vi "dfd_NStage MRate Response with Overall.vi"(4 "interpolated factors":i32[](array[numeric]), 5 "type (FLP)":enum16{"FLP", "FXP"}(ring), 6 "fs [Hz]":dbl, 7 "# freq bins (auto)":i32, 8 "error in (no error)":errorcluster, 9 "magnitude":u16(ring) items=["Linear", "dB", "Zero phase"], 10 "phase view":T1, 11 "multirate filters in":T2[](array[typedef]) {"mMRate_SumWl" min=1 max=32 step=1; "mMRate_InputIwl" min=1 max=32 step=1; "mMRate_GainWl" min=1 max=32 step=1; "mMRate_OutputWl" min=1 max=32 step=1; "mMRate_InputWl" min=1 max=32 step=1; "mMRate_CoefWl" min=1 max=32 step=1; "mMRate_Mode" items=["Default"=-1, "No Rate Change"=0, "Interpolation"=1, "Decimation"=2, "Interpolated"=3, "Rational"=4]}) -> (0 "error out":errorcluster, 2 "phase":cluster{dbl, "df":dbl, "phase":dbl[]}[](array[cluster]), 3 "mag":cluster{dbl, "df":dbl, "magnitude":dbl[]}[](array[cluster]))   [LabVIEW 2017, in "NI_DigFilterLicensed.lvlib"]
uses:
  <vilib>/addons/Digital Filter Design/NI_DigFilterLicensed.lvlib
  <vilib>/addons/Digital Filter Design/_Objects.llb/DFD Multirate Filter Obj.ctl
  <vilib>/addons/Digital Filter Design/_Objects.llb/DFD Multirate Mode.ctl
  <vilib>/addons/Digital Filter Design/_Objects.llb/DFD Coef Norm Type.ctl
  <vilib>/addons/Digital Filter Design/_Objects.llb/DFD Round-off Mode.ctl
  <vilib>/addons/Digital Filter Design/_Objects.llb/DFD FXP MRate Multiply Mode.ctl
  <vilib>/addons/Digital Filter Design/_Objects.llb/DFD Phase Setting.ctl
  <vilib>/Analysis/2dsp.llb/1D Convolution (DBL).vi
  <vilib>/Analysis/NI_AALPro.lvlib
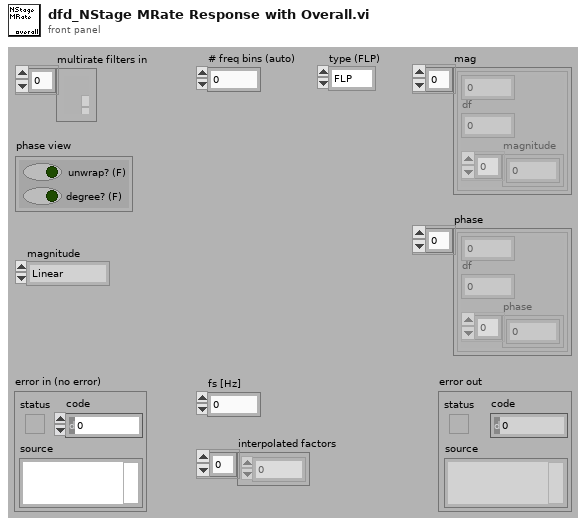
[diagram p1: front panel]
types:
  T1 = typedef "NI_DigFilterLicensed.lvlib/DFD Phase Setting.ctl" = cluster{"unwrap? (F)":bool, "degree? (F)":bool}
  T2 = typedef "NI_DigFilterLicensed.lvlib/DFD Multirate Filter Obj.ctl" = cluster{"mMRate_Structure":enum16{"CIC", "FIR", "IIR", "Lattice"}, "mMRate_Mode":T3, "mMRate_Factor":i32, "mMRate_FIRParams":cluster{"mMRate_FIR_H":dbl[], "mMRate_FIR_IsNyquist?":bool, "mMRate_FIR_IsSymmetric?":bool}, "mMRate_CICParams":cluster{"mMRate_CIC_#Stage":i32, "mMRate_CIC_Lag":i32, "mMRate_CIC_Type":enum16{"Lowpass", "Highpass"}}, "mMRate_Order":i32, "mMRate_Version":string, "mMRate_Comments":string, "mMRate_RationalFactor":cluster{"mMRate_L":i32, "mMRate_M":i32}, "mMRate_Fs":dbl, "mMRate_Quantized?":bool, "mMRate_QFilterGain":dbl, "mMRate_CoefWl":i16, "mMRate_Scaling":cluster{"mMRate_ScaleByPowerOf2?":bool, "mMRate_ScaleType":T4}, "mMRate_InputWl":i16, "mMRate_OutputWl":i16, "mMRate_OutputMode":T5, "mMRate_MultMode":T6, "mMRate_BitPruning":bool, "mMRate_GainWl":i16, "mMRate_OutputFwl":i16, "mMRate_SumIwl":i16, "mMRate_InputIwl ":i16, "mMRate_SumWl":i16, "mMRate_CoefIwl":i16}
  T3 = typedef "NI_DigFilterLicensed.lvlib/DFD Multirate Mode.ctl" = i16
  T4 = typedef "NI_DigFilterLicensed.lvlib/DFD Coef Norm Type.ctl" = enum16{"No Norm", "Time Domain 1-Norm", "Time Domain 2-Norm", "Time Domain Inf-Norm"}
  T5 = typedef "NI_DigFilterLicensed.lvlib/DFD Round-off Mode.ctl" = enum16{"Nearest", "Truncation"}
  T6 = typedef "NI_DigFilterLicensed.lvlib/DFD FXP MRate Multiply Mode.ctl" = enum16{"Truncated", "Full"}
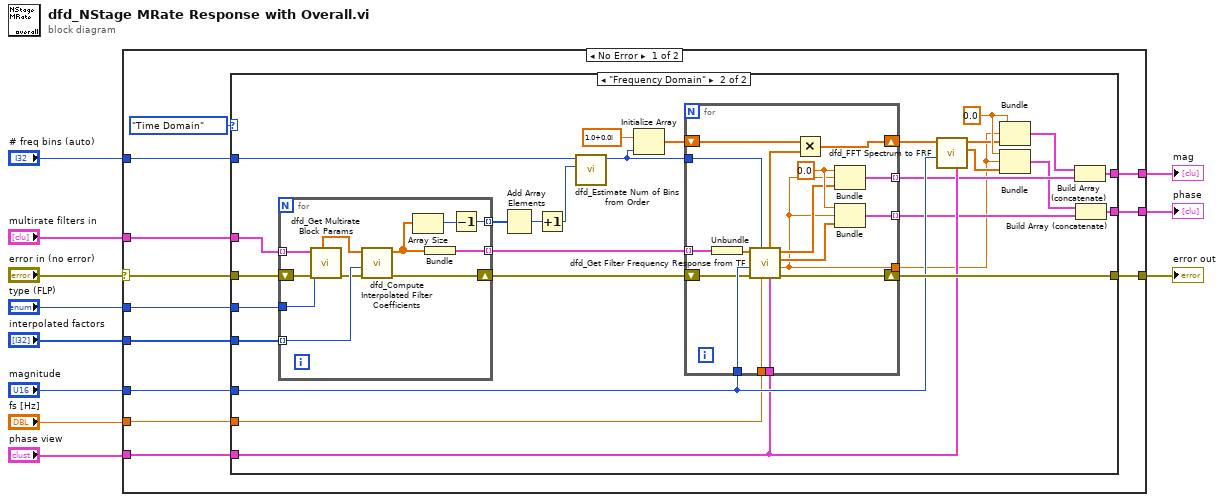
[diagram p0: block diagram]
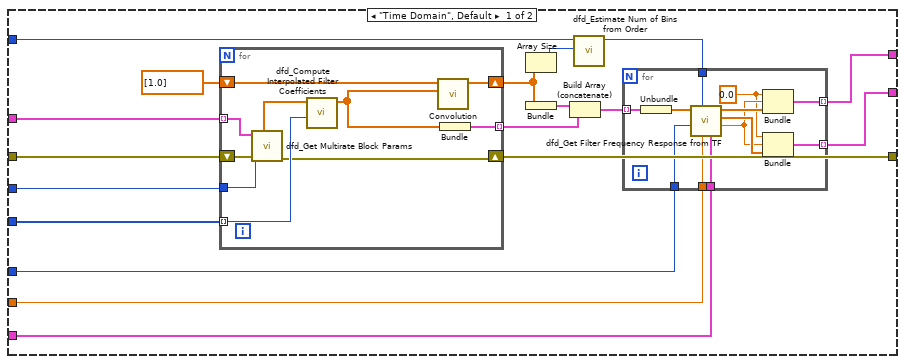
[diagram p2: hidden frame]
diagram:
  n1 = case shown="No Error" "error in (no error)" {
    selector: "error in (no error)" -> [w21 w120]
    tunnel: "multirate filters in" -> [w20 _]
    tunnel: "interpolated factors" -> [w23 _]
    tunnel: "# freq bins (auto)" -> [w22 _]
    tunnel: "fs [Hz]" -> [w13 _]
    tunnel: "magnitude" -> [w17 _]
    tunnel: "phase view" -> [w16 _]
    tunnel: [w18 w120] -> w1
    tunnel: "type (FLP)" -> [w19 _]
    tunnel: [w15 _] -> w3
    tunnel: [w14 _] -> w2
    frame No Error {
      n2 = case shown="\"Frequency Domain\"" enum16{"Time Domain", "Frequency Domain"}."Time Domain" ("Enum") {
        tunnel: w23 -> [w27 w91]
        tunnel: w22 -> [w29 w90]
        tunnel: w21 -> [w31 w89]
        tunnel: w20 -> [w30 w86]
        tunnel: w19 -> [w28 w85]
        tunnel: [w32 w82] -> w18
        tunnel: w17 -> [w26 w80]
        tunnel: w16 -> [w24 w79]
        tunnel: [w34 w72] -> w15
        tunnel: [w33 w71] -> w14
        tunnel: w13 -> [w25 w69]
        frame "Time Domain", Default {
          n3 = for {
            tunnel: w30 -> [w63] mode=indexing
            tunnel: w27 -> [w60] mode=indexing
            shift-right: [w61] -> w37
            shift-left: dbl[] [1.0] -> [w62]
            tunnel: [w58] -> w41 mode=indexing
            tunnel: w28 -> [w56]
            shift-right: [w55] -> w32
            shift-left: w31 -> [w54]
            n4 = call <vilib>:"dfd_Get Multirate Block Params.vi"("error in (no error)"=w54, "type (FLP)"=w56, "multirate filter in"=w63) -> ("error out"=w55:errorcluster, "FIR"=w57:dbl[])  [unwired: 1 in, 6 out]
            n5 = call <vilib>:"dfd_Compute Interpolated Filter Coefficients.vi"("factor"=w60, "numerator in"=w57) -> ("numerator out"=w59:dbl[])  [unwired: 2 in, 7 out]
            n6 = call-poly <vilib>:"Convolution.vi"("Y"=w59, "X"=w62) -> ("X * Y"=w61:dbl[])  [unwired: 1 in, 8 out]
            n7 = Bundle("numerator out"=w59) -> (w58:cluster{"numerator out":dbl[]})  [unwired: 1 in]
          }
          n8 = Array Size(array=w37) -> (size(s)=w36:i32)
          n9 = Bundle(w37) -> (w38:cluster{dbl[]})  [unwired: 1 in]
          n10 = Build Array (concatenate)(w38, w41) -> (w39:cluster{"numerator out":dbl[]}[])
          n11 = call <vilib>:"dfd_Estimate Num of Bins from Order.vi"("order"=w36, "# freq bins in"=w29) -> ("# freq bins out"=w40:i32)  [unwired: 9 out]
          n12 = for {
            tunnel: w39 -> [w53] mode=indexing
            tunnel: w40 -> [w51]
            tunnel: w25 -> [w50]
            tunnel: w26 -> [w49]
            tunnel: w24 -> [w48]
            tunnel: [w43] -> w34 mode=indexing
            tunnel: [w42] -> w33 mode=indexing
            w44 = 0.0
            n13 = Unbundle(w53) -> ("numerator out"=w52:dbl[])
            n14 = call <vilib>:"dfd_Get Filter Frequency Response from TF.vi"("phase view"=w48, "fs [Hz]"=w50, "# freq bins (512)"=w51, "magnitude"=w49, "num"=w52) -> ("df"=w45:dbl, "phase"=w46:dbl[], "magnitude"=w47:dbl[])  [unwired: 2 in, 2 out]
            n15 = Bundle(w44, "df"=w45, "magnitude"=w47) -> (w43:cluster{dbl, "df":dbl, "magnitude":dbl[]})  [unwired: 1 out]
            n16 = Bundle(w44, "df"=w45, "phase"=w46) -> (w42:cluster{dbl, "df":dbl, "phase":dbl[]})  [unwired: 1 out]
          }
        }
        frame "Frequency Domain" {
          w83 = 0.0
          n17 = for {
            tunnel: w86 -> [w119] mode=indexing
            tunnel: w91 -> [w116] mode=indexing
            tunnel: w85 -> [w118]
            shift-right: [w114] -> w84
            shift-left: w89 -> [w117]
            tunnel: [w111] -> w88 mode=indexing
            tunnel: [w109] -> w70 mode=indexing
            n18 = call <vilib>:"dfd_Get Multirate Block Params.vi"("error in (no error)"=w117, "type (FLP)"=w118, "multirate filter in"=w119) -> ("error out"=w115:errorcluster, "FIR"=w113:dbl[])  [unwired: 1 in, 6 out]
            n19 = call <vilib>:"dfd_Compute Interpolated Filter Coefficients.vi"("error in (no error)"=w115, "factor"=w116, "numerator in"=w113) -> ("error out"=w114:errorcluster, "numerator out"=w110:dbl[])  [unwired: 1 in, 6 out]
            n20 = Array Size(array=w110) -> (size(s)=w112:i32)
            n21 = Bundle("numerator out"=w110) -> (w109:cluster{"numerator out":dbl[]})  [unwired: 1 in]
            n22 = Decrement(x=w112) -> (x-1=w111:i32)
          }
          n23 = Add Array Elements(numeric array=w88) -> (sum=w87:i32)
          n24 = Increment(x=w87) -> (x+1=w67:i32)
          n25 = call <vilib>:"dfd_Estimate Num of Bins from Order.vi"("order"=w67, "# freq bins in"=w90) -> ("# freq bins out"=w64:i32)  [unwired: 9 out]
          n26 = Initialize Array(cdb 1.0+0.0i ("element"), w64) -> (w65:cdb[])
          n27 = for {
            tunnel: w64 -> [w108]
            tunnel: w80 -> [w107]
            shift-right: [w103] -> w82
            shift-left: w84 -> [w95]
            shift-right: [w92] -> w81
            shift-left: w65 -> [w106]
            tunnel: w69 -> [w105]
            tunnel: w79 -> [w104]
            tunnel: [w98] -> w75 mode=indexing
            tunnel: [w97] -> w73 mode=indexing
            tunnel: w70 -> [w96] mode=indexing
            tunnel: [w94] -> w68
            w101 = 0.0
            n28 = Unbundle(w96) -> ("numerator out"=w93:dbl[])
            n29 = call <vilib>:"dfd_Get Filter Frequency Response from TF.vi"("phase view"=w104, "fs [Hz]"=w105, "# freq bins (512)"=w108, "error in (no error)"=w95, "magnitude"=w107, "num"=w93) -> ("error out"=w103:errorcluster, "df"=w94:dbl, "phase"=w99:dbl[], "magnitude"=w100:dbl[], "X(w)"=w102:cdb[])  [unwired: 1 in]
            n30 = Multiply(x=w106, y=w102) -> (x*y=w92:cdb[])
            n31 = Bundle(w101, "df"=w94, "magnitude"=w100) -> (w98:cluster{dbl, "df":dbl, "magnitude":dbl[]})  [unwired: 1 out]
            n32 = Bundle(w101, "df"=w94, "phase"=w99) -> (w97:cluster{dbl, "df":dbl, "phase":dbl[]})  [unwired: 1 out]
          }
          n33 = call <vilib>:"dfd_FFT Spectrum to FRF.vi"("phase view"=w79, "magnitude"=w80, "FFT {X}"=w81) -> ("phase"=w77:dbl[], "amplitude"=w78:dbl[])  [unwired: 3 in, 4 out]
          n34 = Bundle(w83, "df"=w68, "amplitude"=w78) -> (w76:cluster{dbl, "df":dbl, "amplitude":dbl[]})  [unwired: 1 out]
          n35 = Bundle(w83, "df"=w68, "phase"=w77) -> (w74:cluster{dbl, "df":dbl, "phase":dbl[]})  [unwired: 1 out]
          n36 = Build Array (concatenate)(w76, w75) -> (w72:cluster{dbl, "df":dbl, "magnitude":dbl[]}[])
          n37 = Build Array (concatenate)(w74, w73) -> (w71:cluster{dbl, "df":dbl, "phase":dbl[]}[])
        }
      }
    }
    frame Error {
    }
  }
  "error out" <- w1
  "phase" <- w2
  "mag" <- w3
